vi "Digital Exposure Controller.vi"(11 "State in":T1) -> (3 "State":T1)   [LabVIEW 2020]
uses:
  CFTS Main Panel SubVIs/CFTS-Experiment State.ctl
  Typedefs/Exposure-Options.ctl
  epl-vi-lib/Signal Synthesis VIs/Top Level VIs/Stimulus-Set Level (array).vi
panel:
  in  "Brickwall":bool caption="Brickwall filter"
  in  "InvFilt":bool caption="Precompensate noise"
  in  "Auto adjust level":bool
  in  "Params":T2={"Probe Mic Gain"=40.0, "Waveform"=enum."Tone", "CF (kHz)"=1.0, "BW (kHz)"=4.0, "Ear"=enum."Left", "Duration (min)"=0.0, "dB SPL (right)"=120.0, "dB SPL 2"=120.0}
  in  "START":bool
  in  "RETURN":bool
  in  "STOP":bool
  out "Log":cluster{dbl, "Buffer length (s)":dbl, dbl[][]}(graph)
  out "update Max SPL":bool
  out "exit signal":bool
  out "Gauge 2":dbl(knob)=99.37258874088361 scale=80.0..130.0
  out "dB SPL rms 2":dbl=99.37258874088361 caption="Left (dB SPL)" format="%.2f"
  out "Max SPL Left":dbl=120.0 caption="Max" format="%.2g"
  in  "Options":T3={"Tracking"={"Tolerance (dB)"=0.25, "T (s)"=3.0}, "Seeds"={"Left"=0, "Right"=0}}
  out "Max SPL":dbl=120.0 caption="Max" format="%.2g"
  out "Abort":bool
  in  "Buffer length (s)":dbl=1.0
  in  "Sampling rate (Hz)":dbl=100000.0
  out "Elapsed time":string
  out "Gauge":dbl(knob)=99.37258874088361 scale=80.0..130.0
  out "dB SPL rms":dbl=99.37258874088361 caption="dB SPL" format="%.2f"
  out "Waveform":waveform(dbl)[](graph)
  out "Spectrum":waveform(dbl)[](graph)
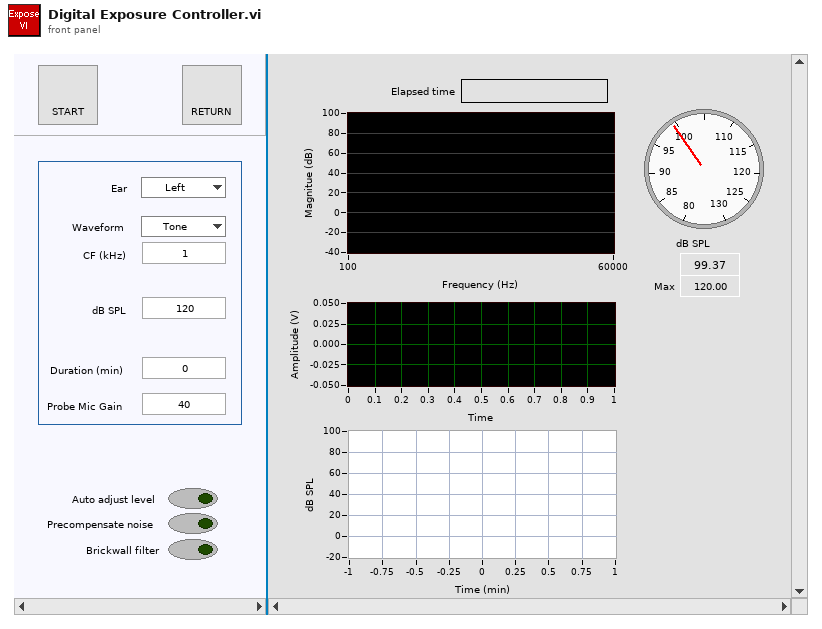
[diagram p1: front panel]
types:
  T1 = typedef "CFTS-Experiment State.ctl" = cluster{"Experimenter":string, "Number":u32, "Right":string, "Left":string, "Data Folder":path, "State File":path, "Version Info":string, "End Exposure Time":dbl, "Exposure Duration":string, "Run #":cluster{"CAP":i16, "ABR":i16, "DP":i16, "VsEP":i16, "MeasSeq":i16, "SubSeq":i16, "SFOAE":i16}}
  T2 = cluster{"Probe Mic Gain":dbl, "Waveform":enum16{"Tone", "Noise"}, "CF (kHz)":dbl, "BW (kHz)":dbl, "Ear":enum16{"Right", "Left", "Binaural"}, "Duration (min)":dbl, "dB SPL (right)":dbl, "dB SPL 2":dbl}
  T3 = typedef "Exposure-Options.ctl" = cluster{"Tracking":cluster{"Tolerance (dB)":dbl, "T (s)":dbl}, "Seeds":cluster{"Left":i32, "Right":i32}}
  T4 = typedef "Exposure-Runtime Data.ctl" = cluster{"Probe Tube Mag":dbl[][], "AI Order":i32[]}
  T5 = typedef "Stimulus Channel.xctl/Stimulus Channel Data.ctl" = cluster{"Waveform":T6, "Filter":T23, "Gate":T24, "Level":T25}
  T6 = typedef "Waveform XCtl.xctl/Waveform Data.ctl" = cluster{"Type":T7, "Tone":T8, "Pulse Train":T9, "Noise":T12, "File":T13, "FMSweep":T14, "Chirp Train":T15, "Complex Tone":cluster{"Params":T17, "Data":T19}, "Moving Ripple":T20}
  T7 = typedef "Waveform Enum.ctl" = enum16{"OFF", "Tone", "Noise", "Pulse Train", "File", "FM Sweep", "Chirp Train", "Complex Tone", "FM Tone", "Moving Ripple"}
  T8 = typedef "Tone Params.ctl" = cluster{"Frequency (kHz)":dbl, "Last Freq":dbl, "Last Phase":dbl}
  T9 = typedef "Pulse Train Params.ctl" = cluster{"Pulse width (us)":dbl, "Pulse rate (Hz)":dbl, "Gap (ms)":dbl, "Polarity":T10, "PT State":T11, "Asynch":bool}
  T10 = typedef "Pulse Polarity.ctl" = enum16{"POS", "NEG", "POS-NEG", "NEG-POS"}
  T11 = typedef "PT-Continuous State.ctl" = cluster{"Template":dbl[], "Nperiod":i32, "Index":i32, "Pulse Rate (Hz)":dbl, "Phase (cycles)":dbl, "Noff":i32}
  T12 = typedef "Noise Params.ctl" = cluster{"InvFilt":bool, "Noise":dbl[], "CurPt":i32, "Aweight":bool, "Seed":i32, "afile":path}
  T13 = typedef "StimFile-Params.ctl" = cluster{"Filename":path, "Signal":dbl[], "Channel":i32, "stream":bool, "offset":i32, "nreps":i32, "loops":i32, "Randomize":bool, "order":i32[], "Seed":i32, "Tokens":i32}
  T14 = typedef "FM Sweep Params.ctl" = cluster{"Rate (oct/s)":dbl, "Fmin (Hz)":dbl, "Fmax (Hz)":dbl, "Ramp (ms)":dbl, "Linear":bool}
  T15 = typedef "Chirp Train.ctl" = cluster{"Params":T16, "Data":cluster{"WF":dbl[]}}
  T16 = typedef "Chirp Train Params.ctl" = cluster{"Fmin (kHz)":dbl, "Fmax (kHz)":dbl, "Compensate":bool, "Duration (ms)":dbl}
  T17 = typedef "CT-Params.ctl" = cluster{"F0 (Hz)":dbl, "Band":cluster{"Flow (Hz)":dbl, "Fhigh (Hz)":dbl}, "Phase":T18, "Min F0 (Hz)":dbl, "Max F0 (Hz)":dbl, "ContinRandPhase":bool, "Max peak factor":dbl, "Max mod depth":dbl, "MinHarmNum":i32, "MaxHarmNum":i32, "Level Mode":enum16{"per component", "overall rms"}, "% jitter":dbl}
  T18 = typedef "CT-Phase Enum.ctl" = enum16{"Cosine", "Random", "Alternating"}
  T19 = typedef "CT-Runtime Data.ctl" = cluster{"Ncomp":i32, "MinHarm":i32, "Phase":dbl[], "Amplitude":dbl[], "Npts/frame":i32, "Last F0":dbl, "Fmin":dbl, "Fmax":dbl, "Lslope":dbl, "randphase":bool, "overall rms":bool, "fmult":dbl[], "jittered":bool}
  T20 = typedef "Moving Ripple.ctl" = cluster{"Params":T21, "Data":T22}
  T21 = typedef "Moving Ripple.Params.ctl" = cluster{"Fmin":dbl, "Fmax":dbl, "Density":dbl, "Velocity":dbl, "Depth":dbl, "Phase":dbl, "Comp/oct":i32}
  T22 = typedef "Moving Ripple.Data.ctl" = cluster{"Freq":dbl[], "A":dbl[], "phase":dbl[], "Phase":dbl}
  T23 = typedef "Filter XCtl.xctl/Filter Data.ctl" = cluster{"CF (kHz)":dbl, "BW (kHz)":dbl, "IIR Filter Cluster":cluster{"filter structure":enum32{"IIR 2nd Order", "IIR 4th Order"}, "Reverse Coefficients":dbl[], "Forward Coefficients":dbl[]}, "Final Filter State":dbl[], "Scale Factor":dbl, "Final Filter State 2":dbl[], "Quadrature":bool, "Type":enum16{"Lowpass", "Highpass", "Bandpass", "Bandstop", "OFF"}}
  T24 = typedef "Gate Control.xctl/Gate Data.ctl" = cluster{"Active":bool, "Delay (ms)":dbl, "Width (ms)":dbl, "Ramp (ms)":dbl}
  T25 = typedef "Level XCtl.xctl/Level Data.ctl" = cluster{"Level":dbl, "Units":T26, "Max":dbl, "Multiplier":dbl, "Cal File":path, "Cal":cluster{"Freq (Hz)":dbl[], "Mag (dB SPL)":dbl[], "Phase (deg)":dbl[]}}
  T26 = typedef "Level Units.ctl" = enum16{"dB atten", "dB SPL", "dB re 1 Vrms", "dB V/Hz½", "mW", "dB HL", "Volts", "dB mW"}
  T27 = typedef "Exposure-Inverse Filter Runtime.ctl" = cluster{"Noise":dbl[], "CurPt":i32, "Active":bool}
  T28 = cluster{"Waveform":T6, "Filter":T23, "Gate":T24, "Level":T25}[]
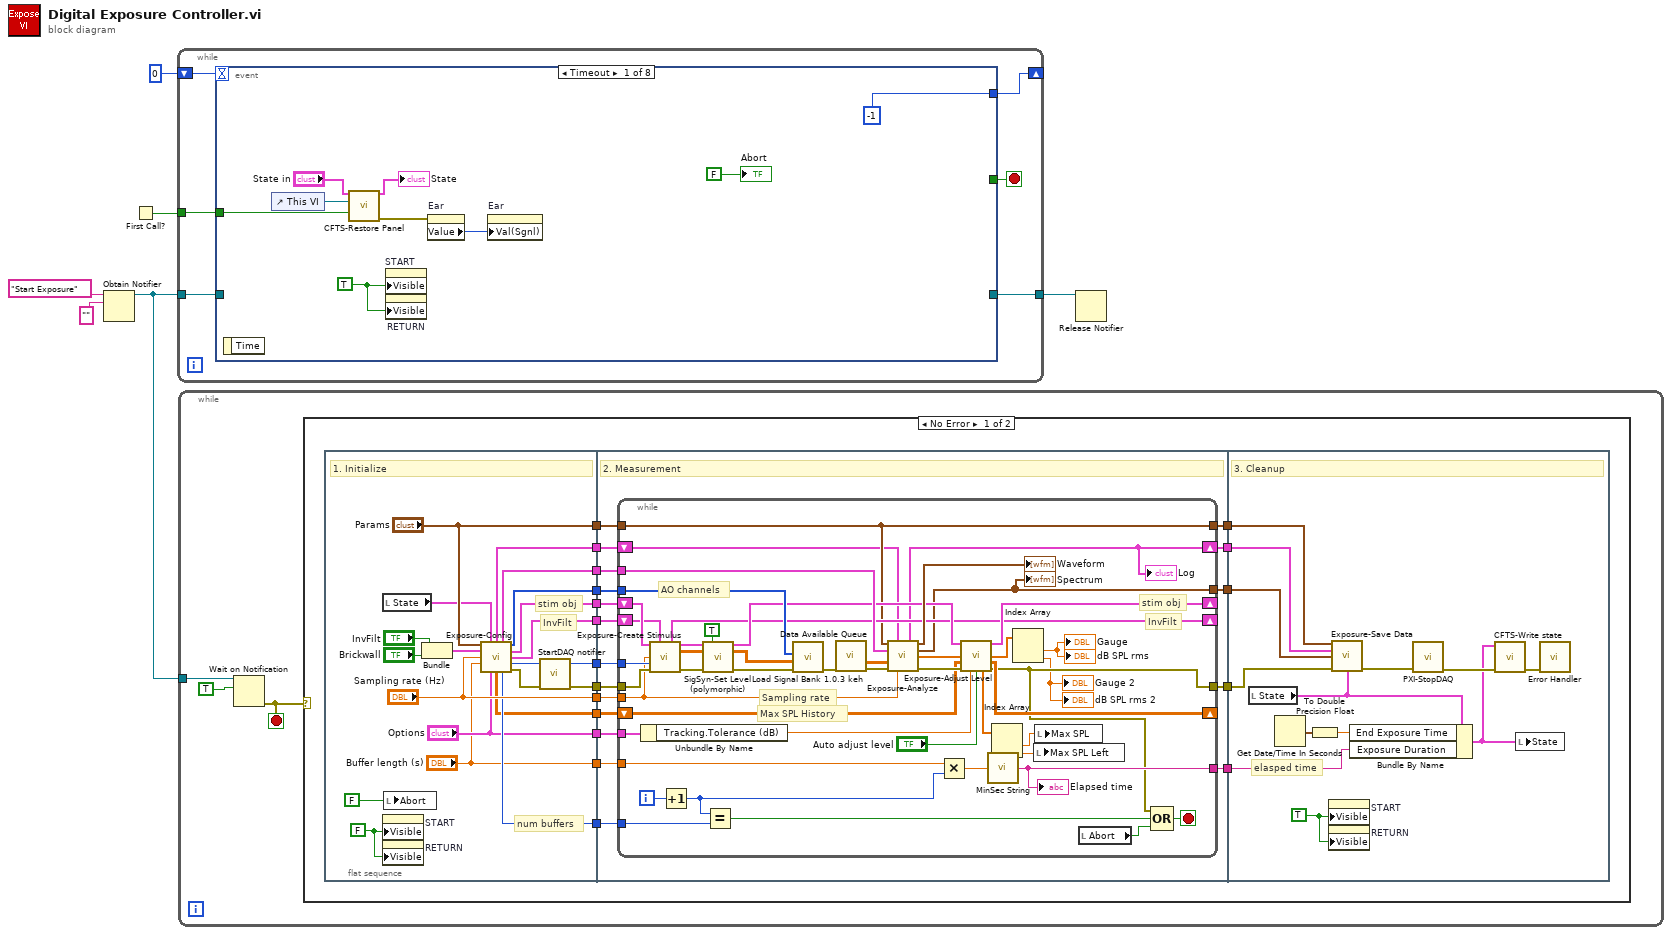
[diagram p0: block diagram]
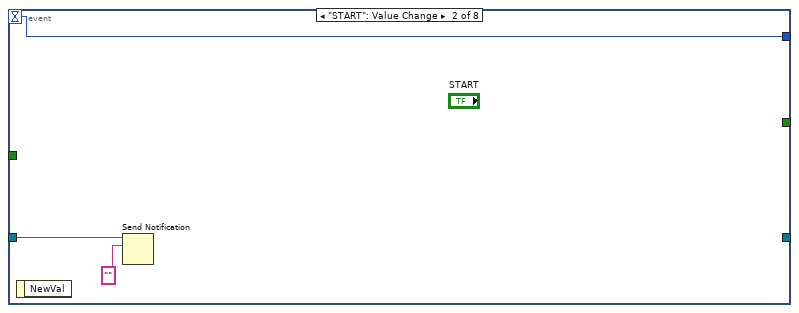
[diagram p3: hidden frame]
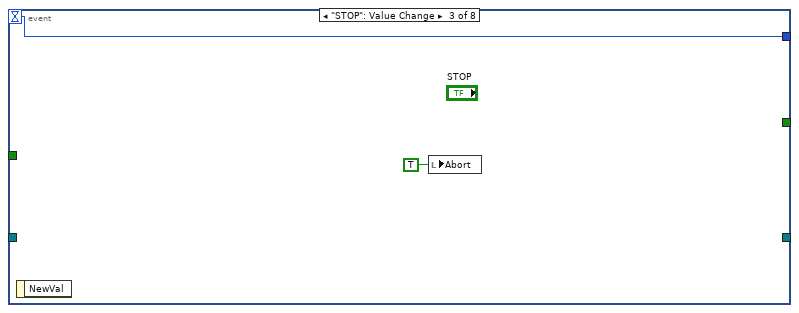
[diagram p4: hidden frame]
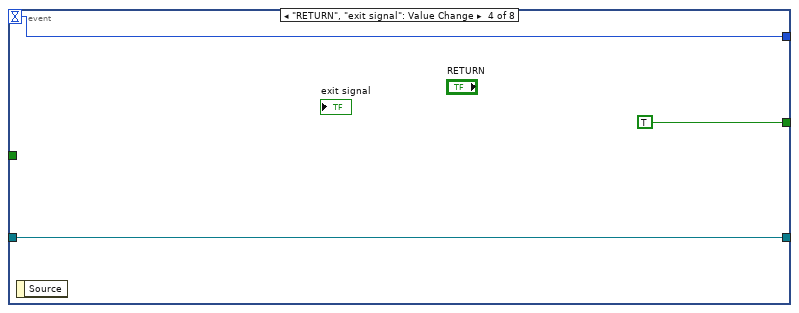
[diagram p5: hidden frame]
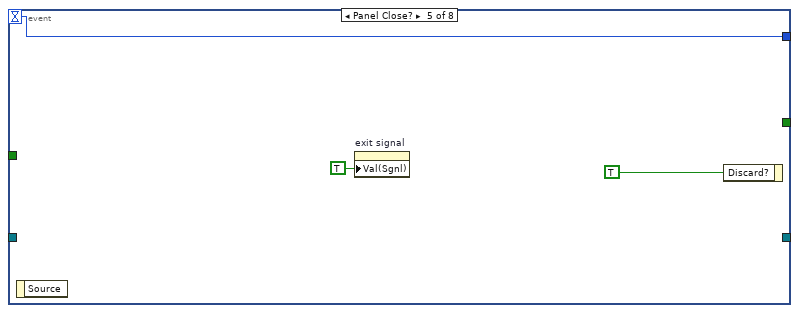
[diagram p6: hidden frame]
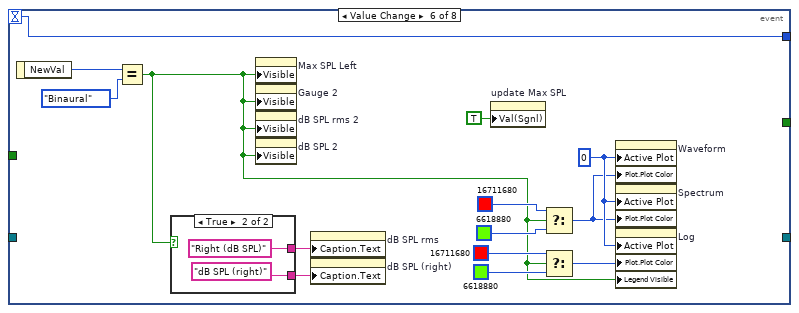
[diagram p7: hidden frame]
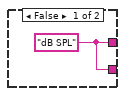
[diagram p8: hidden frame]
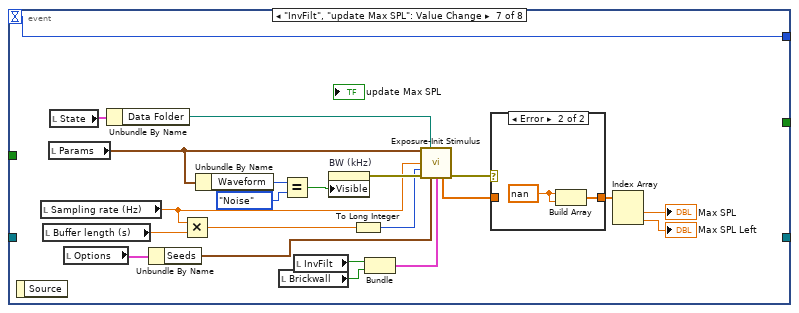
[diagram p9: hidden frame]
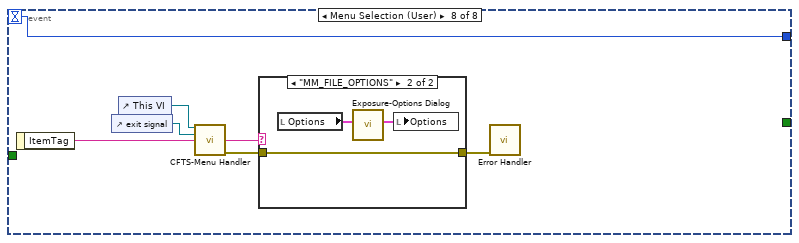
[diagram p11: hidden frame]
diagram:
  n1 = Obtain Notifier(name (unnamed)="Start Exposure", notification data type="") -> (notifier out=w6:refnum<notifier>)  [unwired: 2 in, 2 out]
  n2 = First Call?() -> (First Call?: T/F=w1:bool)
  n3 = while {
    tunnel: w6 -> [w12]
    tunnel: [w10] -> w5
    shift-right: [w8] -> _
    shift-left: 0 -> [w9]
    tunnel: w1 -> [w7]
    stop <- w11 stop-if-true
    n4 = event shown="[0] Timeout" {
      selector: _ -> [_ _ _ _ _ _ _ _]
      dyn-events: _ -> [_ _ _ _ _ _ _ _]
      timeout: w9 -> [_ w22 w25 w27 w32 w46 w71 w78]
      tunnel: w12 -> [_ w23 _ w28 _ _ _ _]
      tunnel: [_ _ _ TRUE _ _ _ _] -> w11
      tunnel: [_ _ _ w28 _ _ _ _] -> w10
      tunnel: [-1 w22 w25 w27 w32 w46 w71 w78] -> w8
      tunnel: w7 -> [w18 _ _ _ _ _ _ _]
      event Timeout {
        w19 = TRUE ("Visible")
        n5 = event-data() -> ()  [unwired: 1 in, 1 out]
        n6 = control-ref of="This VI"() -> (w17:refnum<vi>)
        n7 = call "CFTS-Restore Panel.vi"("State (in)"="State in", "VI refnum"=w17, "Restore?"=w18) -> ("State"=→"State":T1, "error out"=w13:errorcluster)  [unwired: 11 in]
        n8 = property on="START" class="Bool"("Visible"=w19) -> ()  [unwired: 2 in, 2 out]
        n9 = property on="RETURN" class="Bool"("Visible"=w19) -> ()  [unwired: 2 in, 2 out]
        n10 = property on="Ear" class="Enum (strict)"(error in=w13) -> ("Value"=w14:enum16{"Right", "Left", "Binaural"})  [unwired: 1 in, 2 out]
        n11 = property on="Ear" class="Enum (strict)"("Val(Sgnl)"=w14) -> ()  [unwired: 2 in, 2 out]
        "Abort" <- FALSE ("Abort")
      }
      event "START": Value Change {
        n12 = event-data() -> ()  [unwired: 1 in, 1 out]
        n13 = Send Notification(notification="", notifier=w23) -> ()  [unwired: 1 in, 2 out]
      }
      event "STOP": Value Change {
        n14 = event-data() -> ()  [unwired: 1 in, 1 out]
        n15 = local write "Abort"(TRUE ("Global Abort")) -> ()
      }
      event "RETURN", "exit signal": Value Change {
        n16 = event-data() -> ()  [unwired: 1 in, 1 out]
      }
      event Panel Close? {
        n17 = event-data() -> ()  [unwired: 1 in, 1 out]
        n18 = property on="exit signal" class="Bool (strict)"("Val(Sgnl)"=TRUE ("Value (Signaling)")) -> ()  [unwired: 2 in, 2 out]
        n19 = event-data("Discard?"=TRUE) -> ()  [unwired: 1 in, 1 out]
      }
      event "Params.Ear": Value Change {
        w42 = u32 0 ("Active Plot")
        n20 = event-data() -> ("NewVal"=w44:enum16{"Right", "Left", "Binaural"})  [unwired: 1 in]
        n21 = Equal?(x=w44, y=enum16{"Right", "Left", "Binaural"}."Binaural") -> (x = y?=w33:bool)
        n22 = case shown="True" w33 {
          tunnel: [w47 "Right (dB SPL)"] -> w35
          tunnel: [w47 "dB SPL (right)"] -> w34
          frame False {
            w47 = "dB SPL"
          }
          frame True {
          }
        }
        n23 = property on="Max SPL Left" class="DigNum (strict)"("Visible"=w33) -> ()  [unwired: 2 in, 2 out]
        n24 = property on="Gauge 2" class="Knob (strict)"("Visible"=w33) -> ()  [unwired: 2 in, 2 out]
        n25 = property on="dB SPL rms 2" class="DigNum (strict)"("Visible"=w33) -> ()  [unwired: 2 in, 2 out]
        n26 = property on="dB SPL 2" class="DigNum (strict)"("Visible"=w33) -> ()  [unwired: 2 in, 2 out]
        n27 = property on="dB SPL rms" class="DigNum (strict)"("Caption.Text"=w35) -> ()  [unwired: 2 in, 2 out]
        n28 = property on="dB SPL (right)" class="DigNum (strict)"("Caption.Text"=w34) -> ()  [unwired: 2 in, 2 out]
        n29 = property on="update Max SPL" class="Bool (strict)"("Val(Sgnl)"=TRUE ("Value (Signaling)")) -> ()  [unwired: 2 in, 2 out]
        n30 = Select(t=u32 16711680, s=w33, f=u32 6618880) -> (s? t:f=w40:u32)
        n31 = Select(t=u32 16711680, s=w33, f=u32 6618880) -> (s? t:f=w36:u32)
        n32 = property on="Waveform" class="WFGraph (strict)"("Active Plot"=w42, "Plot.Plot Color"=w40) -> ()  [unwired: 2 in, 2 out]
        n33 = property on="Spectrum" class="WFGraph (strict)"("Active Plot"=w42, "Plot.Plot Color"=w40) -> ()  [unwired: 2 in, 2 out]
        n34 = property on="Log" class="WFGraph (strict)"("Active Plot"=w42, "Plot.Plot Color"=w36, "Legend Visible"=w33) -> ()  [unwired: 2 in, 2 out]
      }
      event "Params.Waveform", "Params.CF (kHz)", "Params.BW (kHz)", "InvFilt", "update Max SPL": Value Change {
        n35 = event-data() -> ()  [unwired: 1 in, 1 out]
        n36 = local read "Sampling rate (Hz)"() -> (w62:dbl)
        n37 = local read "Buffer length (s)"() -> (w67:dbl)
        n38 = local read "Params"() -> (w66:T2)
        n39 = local read "State"() -> (w70:T1)
        n40 = local read "Options"() -> (w51:T3)
        n41 = Unbundle By Name(w70) -> ("Data Folder"=w69:path)
        n42 = Unbundle By Name(w51) -> ("Seeds"=w50:cluster{"Left":i32, "Right":i32})
        n43 = Multiply(x=w62, y=w67) -> (x*y=w68:dbl)
        n44 = Unbundle By Name(w66) -> ("Waveform"=w65:enum16{"Tone", "Noise"})
        n45 = local read "Brickwall"() -> (w53:bool)
        n46 = Equal?(x=w65, y=enum16{"Tone", "Noise"}."Noise") -> (x = y?=w58:bool)
        n47 = local read "InvFilt"() -> (w57:bool)
        n48 = property on="BW (kHz)" class="DigNum (strict)"("Visible"=w58) -> (error out=w63:errorcluster)  [unwired: 2 in, 1 out]
        n49 = To Long Integer(number=w68) -> (32bit integer=w59:i32)
        n50 = Bundle("InvFilt"=w57, "Brickwall"=w53) -> (w52:cluster{"InvFilt":bool, "Brickwall":bool})  [unwired: 1 in]
        n51 = call "Exposure-Init Stimulus.vi"("Exposure parameters"=w66, "Data Folder"=w69, "Sampling rate (Hz)"=w62, "Npts"=w59, "error in (no error)"=w63, "Seeds"=w50, "Filter options"=w52) -> ("Max Level"=w60:dbl[], "error out"=w61:errorcluster)  [unwired: 5 in, 2 out]
        n52 = case shown="Error" w61 {
          tunnel: w60 -> [w72 _]
          tunnel: [w72 w74] -> w56
          frame No Error {
          }
          frame Error {
            w73 = nan ("Max Level")
            n53 = Build Array(w73, w73) -> (w74:dbl[])
          }
        }
        n54 = Index Array(array=w56) -> (element #1=→"Max SPL":dbl, element #2=→"Max SPL Left":dbl)  [unwired: 2 in]
      }
      event Menu Selection (User) {
        n55 = event-data() -> ("ItemTag"=w79:string)  [unwired: 1 in]
        n56 = control-ref of="exit signal"() -> (w81:refnum<vi>)
        n57 = control-ref of="This VI"() -> (w80:refnum<vi>)
        n58 = call "CFTS-Menu Handler.vi"("VI Refnum"=w80, "Return Refnum"=w81, "ItemTag"=w79) -> ("ItemTag out"=w75:string, "error out"=w77:errorcluster)  [unwired: 11 in]
        n59 = case shown="\"MM_FILE_OPTIONS\"" w75 {
          tunnel: w77 -> [w82 w85]
          tunnel: [w82 w85] -> w76
          frame "False", Default {
          }
          frame "MM_FILE_OPTIONS" {
            n60 = local read "Options"() -> (w83:T3)
            n61 = call "Exposure-Options Dialog.vi"("Tracking"=w83) -> ("Tracking out"=w84:T3)  [unwired: 9 in, 1 out]
            n62 = local write "Options"(w84) -> ()
          }
        }
        n63 = call "Error Handler.vi"("error in (no error)"=w76) -> ()  [unwired: 13 in, 2 out]
      }
    }
  }
  n64 = while {
    tunnel: w6 -> [w87]
    stop <- w86 stop-if-true
    n65 = Wait on Notification(notifier=w87, ignore previous (F)=TRUE) -> (error out=w86:errorcluster)  [unwired: 2 in, 3 out]
    n66 = case shown="No Error" w86 {
      frame No Error {
        n67 = flat-sequence {
          tunnel: [w125] -> w106
          tunnel: [w114] -> w105
          tunnel: ["Sampling rate (Hz)"] -> w104
          tunnel: [w123] -> w103
          tunnel: [w113] -> w102
          tunnel: [w112] -> w101
          tunnel: ["Buffer length (s)"] -> w100
          tunnel: ["Params"] -> w98
          tunnel: [w111] -> w96
          tunnel: [w118] -> w95
          tunnel: ["Options"] -> w94
          tunnel: [w115] -> w93
          tunnel: [w110] -> w91
          tunnel: w106 -> [w143]
          tunnel: w105 -> [w144]
          tunnel: w104 -> [w142]
          tunnel: w103 -> [w141]
          tunnel: w102 -> [w140]
          tunnel: w101 -> [w139]
          tunnel: w100 -> [w138]
          tunnel: [w137] -> w99
          tunnel: w98 -> [w136]
          tunnel: [w135] -> w97
          tunnel: w96 -> [w134]
          tunnel: w95 -> [w133]
          tunnel: w94 -> [w132]
          tunnel: w93 -> [w131]
          tunnel: [w130] -> w92
          tunnel: w91 -> [w129]
          tunnel: [w128] -> w90
          tunnel: [w127] -> w89
          tunnel: w99 -> [w204]
          tunnel: w97 -> [w201]
          tunnel: w92 -> [w195]
          tunnel: w90 -> [w194]
          tunnel: w89 -> [w192]
          frame #0 {
            w121 = FALSE ("Visible")
            # "InvFilt"
            # "stim obj"
            # "num buffers"
            # "1. Initialize"
            n68 = local read "State"() -> (w120:T1)
            n69 = property on="START" class="Bool"("Visible"=w121) -> ()  [unwired: 2 in, 2 out]
            n70 = property on="RETURN" class="Bool"("Visible"=w121) -> ()  [unwired: 2 in, 2 out]
            n71 = local write "Abort"(FALSE ("Global Abort")) -> ()
            n72 = Bundle("InvFilt"="InvFilt", "Brickwall"="Brickwall") -> (w107:cluster{"InvFilt":bool, "Brickwall":bool})  [unwired: 1 in]
            n73 = call "Exposure-Config.vi"("Exposure parameters"="Params", "Expt State"=w120, "Filter options"=w107, "Sampling rate (Hz)"="Sampling rate (Hz)", "Buffer length (s)"="Buffer length (s)", "Options"="Options") -> ("SPL Log"=w110:cluster{dbl, "Buffer length (s)":dbl, dbl[][]}, "Runtime"=w111:T4, "AO Channels"=w112:i32[], "stimulus"=w114:T5[], "InvFilt"=w115:T27[], "Npts"=w113:i32, "Max SPL History"=w118:dbl[][], "Num Buffers"=w123:i32, "error out"=w126:errorcluster)  [unwired: 1 in]
            n74 = call "StartDAQ notifier.vi"("error in (no error)"=w126) -> ("error out"=w125:errorcluster)  [unwired: 6 in]
          }
          frame #1 {
            # "2. Measurement"
            n75 = while {
              shift-right: [w172] -> _
              shift-left: w144 -> [w176]
              tunnel: w142 -> [w162]
              tunnel: w141 -> [w187]
              tunnel: w140 -> [w190]
              tunnel: w139 -> [w188]
              tunnel: w138 -> [w181]
              tunnel: w136 -> [w150]
              tunnel: [w177] -> w135
              tunnel: w134 -> [w178]
              shift-right: [w169] -> _
              shift-left: w133 -> [w170]
              tunnel: w132 -> [w168]
              shift-right: [w164] -> _
              shift-left: w131 -> [w165]
              tunnel: [w150] -> w130
              shift-right: [w146] -> w128
              shift-left: w129 -> [w147]
              tunnel: [w145] -> w127
              tunnel: w143 -> [w191]
              tunnel: [w163] -> w137
              i -> [w148]
              stop <- w185 stop-if-true
              # "InvFilt"
              # "Max SPL History"
              # "stim obj"
              # "AO channels"
              # "Sampling rate"
              n76 = Unbundle By Name(w168) -> ("Tracking.Tolerance (dB)"=w166:dbl)
              n77 = call "Exposure-Create Stimulus.vi"("StimChan In"=w176, "InvFilt In"=w165, "Sampling rate (Hz)"=w162, "Npts"=w190, "error in (no error)"=w191) -> ("InvFilt Out"=w164:T27[], "StimChan Out"=w160:T5[], "Stimulus"=w159:dbl[][], "error out"=w180:errorcluster)  [unwired: 7 in]
              n78 = Increment(x=w148) -> (x+1=w149:i32)
              n79 = call-poly "SigSyn-Set Level (polymorphic).vi"("AO Control in"=w160, "Apply multiplier? (F)"=TRUE ("Apply multiplier?"), "Waveform in"=w159, "error in (no error)"=w180) -> ("AO Control out"=w173:T28, "Waveform out"=w161:dbl[][], "error out"=w179:errorcluster)  [unwired: 6 in, 3 out]
              n80 = Equal?(x=w149, y=w187) -> (x = y?=w186:bool)
              n81 = call "Load Signal Bank 1.0.3 keh.vi"("error in (no error)"=w179, "Input array"=w161, "Active AO Array"=w188) -> ("error out"=w189:errorcluster)  [unwired: 6 in, 2 out]
              n82 = call "Data Available Queue.vi"("error in (no error)"=w189) -> ("AI Waveforms"=w183:dbl[][], "error out"=w184:errorcluster)  [unwired: 10 in, 3 out]
              n83 = call "Exposure-Analyze.vi"("Exposure parameters"=w150, "SPL Log In"=w147, "Runtime Data"=w178, "AI Waveforms"=w183, "error in (no error)"=w184, "Sampling Rate (Hz)"=w162) -> ("SPL Log Out"=w146:cluster{dbl, "Buffer length (s)":dbl, dbl[][]}, "Waveform"=→"Waveform":waveform(dbl)[], "Spectrum"=w145:waveform(dbl)[], "PT SPL"=w171:dbl[], "error out"=w174:errorcluster)  [unwired: 5 in]
              "Spectrum" <- w145
              "Log" <- w146
              n84 = Multiply(x=w181, y=w149) -> (x*y=w151:dbl)
              n85 = call "Exposure-Adjust Level.vi"("Stimulus In"=w173, "Meas SPL"=w171, "Max SPL History"=w170, "error in (no error)"=w174, "Tolerance (dB)"=w166, "Adjust?"="Auto adjust level") -> ("Stimulus Out"=w172:T5[], "Meas SPL thru"=w154:dbl[], "Max SPL History out"=w169:dbl[][], "Max SPL"=w156:dbl[], "error out"=w163:errorcluster)  [unwired: 5 in]
              n86 = call "MinSec String.vi"("Seconds"=w151) -> ("MinSec string"=w177:string)
              "Elapsed time" <- w177
              n87 = Index Array(array=w156) -> (element #1=w157:dbl, element #2=w155:dbl)  [unwired: 2 in]
              n88 = Index Array(array=w154) -> (element #1=→"Gauge" →"dB SPL rms":dbl, element #2=→"Gauge 2" →"dB SPL rms 2":dbl)  [unwired: 2 in]
              n89 = local write "Max SPL Left"(w155) -> ()
              n90 = local write "Max SPL"(w157) -> ()
              n91 = local read "Abort"() -> (w175:bool)
              n92 = Compound Arithmetic op=OR(w163, w186, w175) -> (w185:bool)
            }
          }
          frame #2 {
            w202 = TRUE ("Visible")
            # "elasped time"
            # "3. Cleanup"
            n93 = local read "State"() -> (w193:T1)
            n94 = Get Date/Time In Seconds() -> (seconds since 1Jan1904=w203:timestamp)
            n95 = To Double Precision Float(number=w203) -> (double precision float=w200:dbl)
            n96 = property on="START" class="Bool"("Visible"=w202) -> ()  [unwired: 2 in, 2 out]
            n97 = property on="RETURN" class="Bool"("Visible"=w202) -> ()  [unwired: 2 in, 2 out]
            n98 = call "Exposure-Save Data.vi"("Params"=w195, "SPL Log In"=w194, "Spectrum"=w192, "error in (no error)"=w204, "State"=w193) -> ("error out"=w196:errorcluster)  [unwired: 10 in]
            n99 = Bundle By Name(cluster=w193, "End Exposure Time"=w200, "Exposure Duration"=w201) -> (w198:T1)
            n100 = call "PXI-StopDAQ.vi"("error in (no error)"=w196) -> ("error out"=w199:errorcluster)  [unwired: 6 in]
            n101 = call "CFTS-Write state.vi"("error in (no error)"=w199, "Experiment info"=w198) -> ("error out"=w197:errorcluster)  [unwired: 9 in]
            n102 = local write "State"(w198) -> ()
            n103 = call "Error Handler.vi"("error in (no error)"=w197) -> ()  [unwired: 13 in, 2 out]
          }
        }
      }
      frame Error {
      }
    }
  }
  n104 = Release Notifier(notifier=w5) -> ()  [unwired: 2 in, 3 out]
